vi "Output.vi"(6 "Msg Attributes in":refnum<data-value>, 7 "Actor in":refnum<class "Actor.lvclass">, 8 "Error in":errorcluster) -> (0 "Error out":errorcluster, 4 "Msg Attributes out":refnum<data-value>, 5 "Actor out":refnum<class "Actor.lvclass">)   [LabVIEW 2020, in "_Template.lvlib" / "Templates.lvlib" / "TEMPLATE jettl Msg.lvlib" / "TEMPLATE Msg Output.lvclass"]
uses:
  TEMPLATE Msg Output.lvclass
  TEMPLATE Msg Output.lvclass/TEMPLATE Msg Output.ctl
  TEMPLATE jettl Msg/TEMPLATE jettl Msg.lvclass
  jettl/jettl/Actor/Actor.lvclass
  jettl/jettl/Relation.ctl
  jettl/jettl/jettl.lvlib
  jettl/jettl/Teller.ctl
  jettl/jettl/Msg Input/Msg Input.lvclass
  jettl/jettl/Msg Attributes.ctl
  jettl/jettl/Msg Output/Msg Output.lvclass
  jettl/jettl/Msg/Msg.lvclass
  jettl/jettl/Transport/Transport.lvclass
  jettl/jettl/Msgs.ctl
  jettl/jettl/Unified Layer.ctl
  jettl/jettl/Actor Attributes.ctl
panel:
  # "This front panel should not be manipulated."
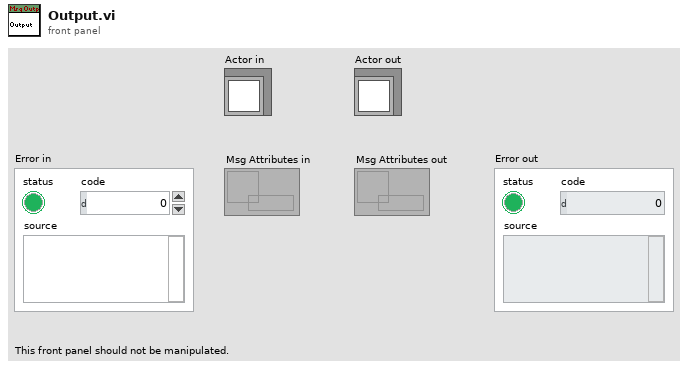
[diagram p1: front panel]
types:
  T1 = typedef "jettl.lvlib/Msg Attributes.ctl" = cluster{"Msg":refnum<class "Msg.lvclass">, "Msg Input":refnum<class "Msg Input.lvclass">, "Msg Output":refnum<class "Msg Output.lvclass">, "Teller":refnum<data-value>}
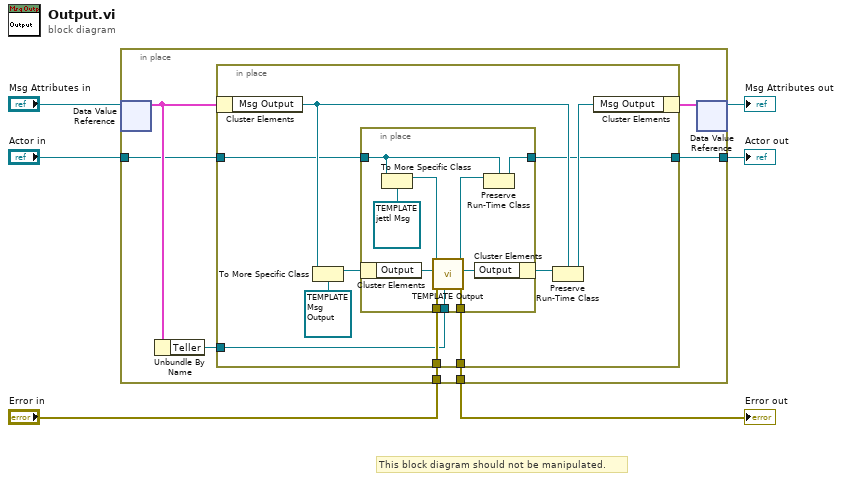
[diagram p0: block diagram]
diagram:
  # "This block diagram should not be manipulated."
  n1 = in-place {
    in-place-border: "Error in" -> [w13]
    in-place-border: [w12] -> w4
    in-place-border: "Actor in" -> [w8]
    in-place-border: [w7] -> w1
    n2 = in-place-dvr #1("Msg Attributes in") -> (w10:T1)  [unwired: 1 out]
    n3 = Unbundle By Name(w10) -> ("Teller"=w9:refnum<data-value>)
    n4 = in-place {
      in-place-border: w13 -> [w23]
      in-place-border: [w22] -> w12
      in-place-border: w9 -> [w17]
      in-place-border: w8 -> [w16]
      in-place-border: [w15] -> w7
      n5 = in-place-cluster #2(w10) -> ("Msg Output"=w20:refnum<class "Msg Output.lvclass">)
      n6 = To More Specific Class(target class=refnum<class "TEMPLATE Msg Output.lvclass"> refnum ("_Template.lvlib:Templates.lvlib:TEMPLATE jettl Msg.lvlib:TEMPLATE Msg Output.lvlib:TEMPLATE Msg Output.lvclass"), reference=w20) -> (specific class reference=w21:refnum<class "TEMPLATE Msg Output.lvclass">)  [unwired: 1 in, 1 out]
      n7 = in-place {
        in-place-border: w23 -> [w28]
        in-place-border: [w27] -> w22
        in-place-border: w17 -> [w26]
        in-place-border: w16 -> [w31]
        in-place-border: [w32] -> w15
        n8 = in-place-cluster #3(w21) -> ("Output"=w30:refnum<data-value>)
        n9 = To More Specific Class(target class=refnum<class "TEMPLATE jettl Msg.lvclass"> refnum ("_Template.lvlib:Templates.lvlib:TEMPLATE jettl Msg.lvlib:TEMPLATE jettl Msg.lvclass"), reference=w31) -> (specific class reference=w25:refnum<class "TEMPLATE jettl Msg.lvclass">)  [unwired: 1 in, 1 out]
        n10 = call-dynamic "TEMPLATE Output.vi"("Teller"=w26, "Error in"=w28, "Output in"=w30, "TEMPLATE jettl Msg in"=w25) -> ("Error out"=w27:errorcluster, "Output out"=w29:refnum<data-value>, "TEMPLATE jettl Msg out"=w24:refnum<class "TEMPLATE jettl Msg.lvclass">)  [unwired: 5 in]
        n11 = in-place-cluster #3("Output"=w29) -> (w19:refnum<class "TEMPLATE Msg Output.lvclass">)
        n12 = Preserve Run-Time Class(object in=w24, 2:w31) -> (object out=w32:refnum<class "Actor.lvclass">)  [unwired: 1 in, 1 out]
      }
      n13 = Preserve Run-Time Class(object in=w19, 2:w20) -> (object out=w18:refnum<class "Msg Output.lvclass">)  [unwired: 1 in, 1 out]
      n14 = in-place-cluster #2("Msg Output"=w18) -> (w11:T1)
    }
    n15 = in-place-dvr #1(w11) -> (→"Msg Attributes out":refnum<data-value>)  [unwired: 1 out]
  }
  "Actor out" <- w1
  "Error out" <- w4
